vi "Read LoopConfig.lvclass.vi"(8 "error in (no error)":errorcluster, 11 "LoopTimer in":refnum<class "LoopTimer.lvclass">) -> (0 "error out":errorcluster, 2 "LoopConfig.lvclass":refnum<class "LoopConfig.lvclass">, 3 "LoopTimer out":refnum<class "LoopTimer.lvclass">)   [LabVIEW 2013, in "ComponentData.lvlib" / "LoopTimer.lvclass"]
uses:
  <userlib>/Common/Component/Application/RT/ComponentData/LoopTimer/LoopTimer.lvclass
  <userlib>/Common/Component/Application/RT/ComponentData/ConfigurationHandler/LoopConfig/LoopConfig.lvclass
  <userlib>/Common/Component/Application/RT/ComponentData/LoopTimer/LoopTimer.lvclass/LoopTimer.ctl
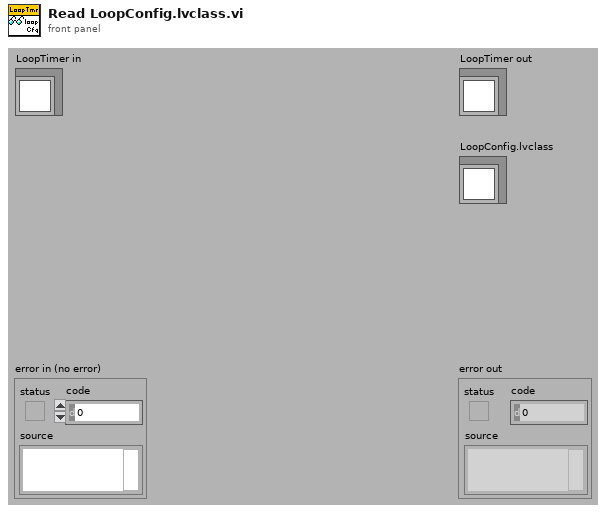
[diagram p1: front panel]
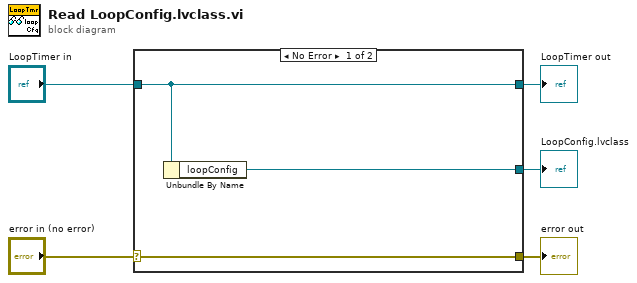
[diagram p0: block diagram]
diagram:
  n1 = case shown="No Error" "error in (no error)" {
    selector: "error in (no error)" -> [w8 w9]
    tunnel: [w8 w9] -> w4
    tunnel: [w7 w10] -> w2
    tunnel: "LoopTimer in" -> [w7 w10]
    tunnel: [w6 _] -> w1
    frame No Error {
      n2 = Unbundle By Name(w7) -> ("loopConfig"=w6:refnum<class "LoopConfig.lvclass">)
    }
    frame Error {
    }
  }
  "error out" <- w4
  "LoopTimer out" <- w2
  "LoopConfig.lvclass" <- w1
